vi "UI.vi"(8 "error in (no error)":errorcluster, 11 "LV Client in":refnum<class "LV Client.lvclass">) -> (0 "error out":errorcluster, 3 "LV Client out":refnum<class "LV Client.lvclass">)   [LabVIEW 2020, in "LV Client.lvclass"]
uses:
  LV Client.lvclass
  LV Client.lvclass/LV Client.ctl
  Common/Message ID.ctl
  <vilib>/IlluminatedG/lv-stream/stream/Stream.lvclass/Stream.ctl
  6d36ac7e-08e4-461e-889e-e636d2d7f3af.vi
  dde1821b-28c5-49a1-9e5e-5f7f2c0cfe74.vi
  1e69932d-3c8f-4f49-a7e3-ed28adad072b.vi
  a13a9a93-203f-4052-94c7-011b74cf2050.vi
  864c4c74-c369-4426-9347-b8c971097d82.vi
  93ec7029-2cc6-4bcf-b00f-f8eb3cee3c3b.vi
  dde1821b-28c5-49a1-9e5e-5f7f2c0cfe74.vi/2114ae84-1210-427f-82ef-c9e9e7f82752.vi
  <vilib>/IlluminatedG/lv-msg-simple/Stream-Simple-Msg/Endpoint/Write Flattened Data.vi
  a13a9a93-203f-4052-94c7-011b74cf2050.vi/2114ae84-1210-427f-82ef-c9e9e7f82752.vi
  93ec7029-2cc6-4bcf-b00f-f8eb3cee3c3b.vi/2114ae84-1210-427f-82ef-c9e9e7f82752.vi
  dde1821b-28c5-49a1-9e5e-5f7f2c0cfe74.vi/2114ae84-1210-427f-82ef-c9e9e7f82752.vi/850aaa44-16cf-4b05-95d8-204edf60ad4b.vi
  <vilib>/IlluminatedG/lv-stream/stream/Write Data.vi
  a13a9a93-203f-4052-94c7-011b74cf2050.vi/2114ae84-1210-427f-82ef-c9e9e7f82752.vi/850aaa44-16cf-4b05-95d8-204edf60ad4b.vi
  93ec7029-2cc6-4bcf-b00f-f8eb3cee3c3b.vi/2114ae84-1210-427f-82ef-c9e9e7f82752.vi/850aaa44-16cf-4b05-95d8-204edf60ad4b.vi
  <vilib>/IlluminatedG/lv-stream/stream/Dispatch Sniffer Data.vi
  <vilib>/IlluminatedG/lv-stream/stream/Prepared.vi
  <vilib>/IlluminatedG/lv-stream/Endpoint/Cast Sniffer Callback.vi
  <vilib>/IlluminatedG/lv-msg-simple/Stream-Simple-Msg/Manager/Endpoints and Formats.vi
  <vilib>/IlluminatedG/lv-msg-simple/Stream-Simple-Msg/Endpoint/Get Format.vi
  <vilib>/IlluminatedG/lv-msg-simple/Stream-Simple-Msg/Endpoint/Get Stream.vi
  <vilib>/Utility/error.llb/Error Cluster From Error Code.vi
  <vilib>/IlluminatedG/lv-stream/stream/Stream.lvclass
  Common/Common.lvlib
panel:
  in  "Reset":bool
  in  "Pause":bool
  in  "Start":bool
  out "State":string
  out "Timer":string
  out "Status":string
  # "Close the window to stop the client."
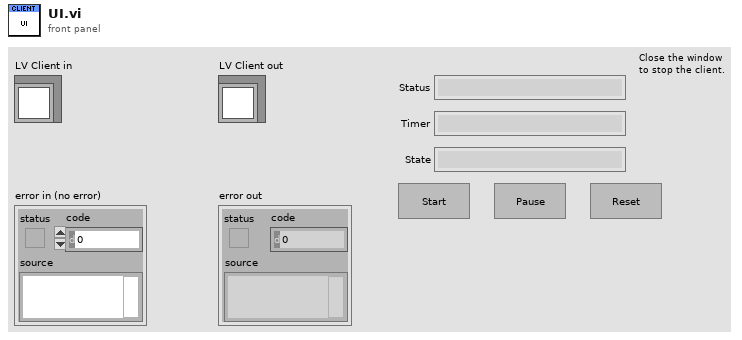
[diagram p1: front panel]
types:
  T1 = typedef "Common.lvlib/Message ID.ctl" = enum16{"Timer State", "Timer Value", "Timer Start", "Timer Pause", "Timer Reset", "Timer Init"}
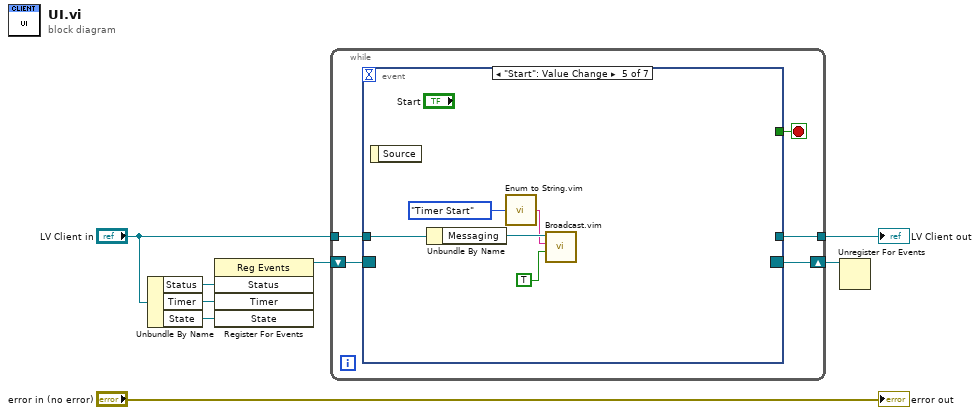
[diagram p0: block diagram]
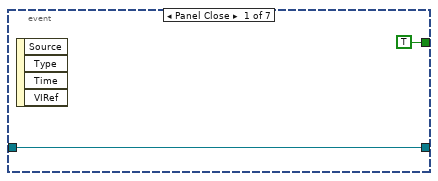
[diagram p2: hidden frame]
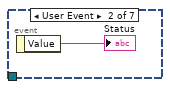
[diagram p3: hidden frame]
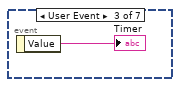
[diagram p4: hidden frame]
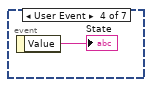
[diagram p5: hidden frame]
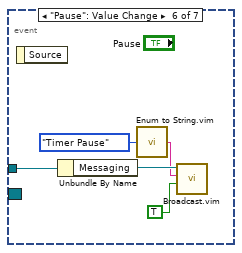
[diagram p6: hidden frame]
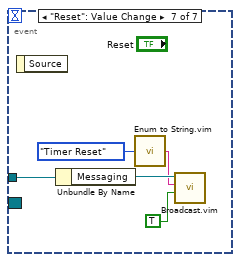
[diagram p7: hidden frame]
diagram:
  n1 = Unbundle By Name("LV Client in") -> ("Status"=w5:refnum<user-event>, "Timer"=w4:refnum<user-event>, "State"=w3:refnum<user-event>)
  n2 = register-events(w5, w4, w3) -> (reference out=w2:refnum<event-registration>)  [unwired: 2 in, 1 out]
  n3 = while {
    tunnel: "LV Client in" -> [w13]
    tunnel: [w11] -> w7
    shift-right: [w9] -> w1
    shift-left: w2 -> [w10]
    stop <- w12 stop-if-true
    n4 = event shown="[4] \"Start\": Value Change" {
      selector: w10 -> [_ _ _ _ _ _ _]
      dyn-events: [_ _ _ _ _ _ _] -> w9
      timeout: _ -> [_ _ _ _ _ _ _]
      tunnel: w13 -> [w14 _ _ _ w19 w24 w33]
      tunnel: [TRUE _ _ _ _ _ _] -> w12
      tunnel: [w14 _ _ _ _ _ _] -> w11
      event Panel Close {
        n5 = event-data() -> ()  [unwired: 1 in, 4 out]
      }
      event User Event {
        n6 = event-data() -> ("Value"=→"Status":string)  [unwired: 1 in]
      }
      event User Event {
        n7 = event-data() -> ("Value"=→"Timer":string)  [unwired: 1 in]
      }
      event User Event {
        n8 = event-data() -> ("Value"=→"State":string)  [unwired: 1 in]
      }
      event "Start": Value Change {
        n9 = event-data() -> ()  [unwired: 1 in, 1 out]
        n10 = Unbundle By Name(w19) -> ("Messaging"=w23:refnum<class "Manager.lvclass">)
        n11 = call "Enum to String.vim"("Enum"=Message_ID."Timer Start" ("Message ID")) -> ("Enum String"=w21:string)
        n12 = call "Broadcast.vim"("Data"=TRUE, "ID"=w21, "Manager in"=w23) -> ()  [unwired: 7 in, 2 out]
      }
      event "Pause": Value Change {
        n13 = event-data() -> ()  [unwired: 1 in, 1 out]
        n14 = Unbundle By Name(w24) -> ("Messaging"=w28:refnum<class "Manager.lvclass">)
        n15 = call "Enum to String.vim"("Enum"=Message_ID."Timer Pause" ("Message ID")) -> ("Enum String"=w26:string)
        n16 = call "Broadcast.vim"("Data"=TRUE, "ID"=w26, "Manager in"=w28) -> ()  [unwired: 7 in, 2 out]
      }
      event "Reset": Value Change {
        n17 = event-data() -> ()  [unwired: 1 in, 1 out]
        n18 = Unbundle By Name(w33) -> ("Messaging"=w32:refnum<class "Manager.lvclass">)
        n19 = call "Enum to String.vim"("Enum"=Message_ID."Timer Reset" ("Message ID")) -> ("Enum String"=w30:string)
        n20 = call "Broadcast.vim"("Data"=TRUE, "ID"=w30, "Manager in"=w32) -> ()  [unwired: 7 in, 2 out]
      }
    }
  }
  "LV Client out" <- w7
  n21 = Unregister For Events(event registration refnum=w1) -> ()  [unwired: 1 in, 1 out]
  "error out" <- "error in (no error)"
